vi "ke37xx Channel Write.vi"(0 "VISA Resource Name":refnum<visa-resource-name>, 5 "Channel":string, 7 "Data (0)":string="0", 9 "Width (1)":string="1", 11 "error in (no error)":errorcluster) -> (4 "VISA Resource Name Out":refnum<visa-resource-name>, 15 "error out":errorcluster)   [LabVIEW 2009, in "Keithley 3700 Series.lvlib"]
doc: "This VI provides a way to write data to Digital I/O, Totalizer and DAC channels."
uses:
  <instrlib>/Keithley 3706/Keithley 3700 Series.lvlib
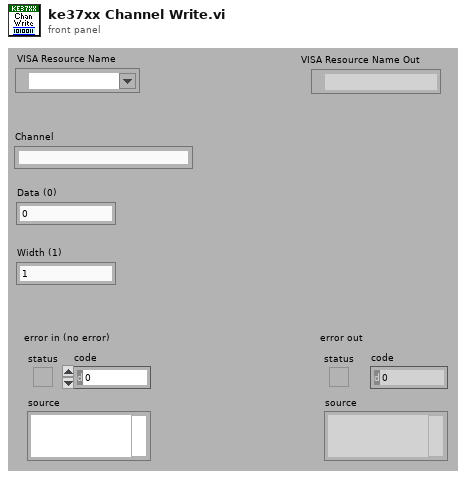
[diagram p1: front panel]
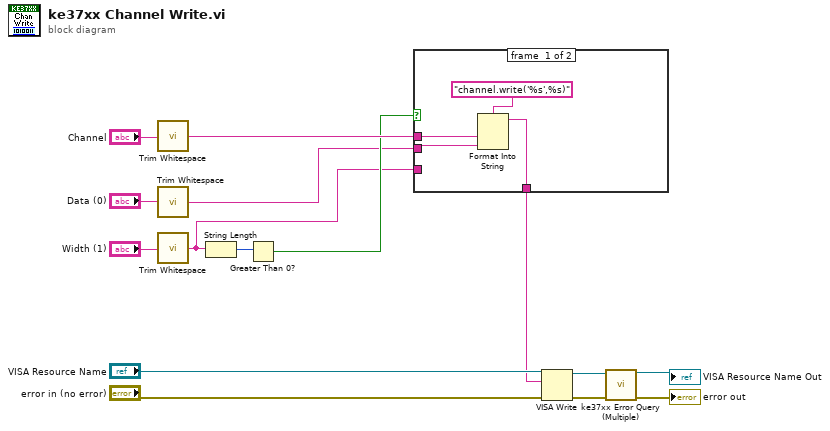
[diagram p0: block diagram]
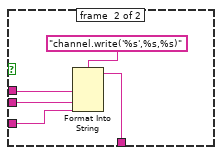
[diagram p2: hidden frame]
diagram:
  n1 = call <vilib>:"Trim Whitespace.vi"("string"="Channel") -> ("trimmed string"=w9:string)  [unwired: 1 in]
  n2 = call <vilib>:"Trim Whitespace.vi"("string"="Data (0)") -> ("trimmed string"=w2:string)  [unwired: 1 in]
  n3 = call <vilib>:"Trim Whitespace.vi"("string"="Width (1)") -> ("trimmed string"=w1:string)  [unwired: 1 in]
  n4 = String Length(string=w1) -> (length=w6:i32)
  n5 = Greater Than 0?(x=w6) -> (x > 0?=w4:bool)
  n6 = case shown="False" w4 {
    tunnel: [w18 w22] -> w11
    tunnel: w9 -> [w17 w23]
    tunnel: w2 -> [w16 w21]
    tunnel: w1 -> [_ w20]
    frame #0 {
      n7 = Format Into String(format string="channel.write('%s',%s)", w17, w16) -> (resulting string=w18:string)  [unwired: 2 in, 1 out]
    }
    frame #1 {
      n8 = Format Into String(format string="channel.write('%s',%s,%s)", w23, w21, w20) -> (resulting string=w22:string)  [unwired: 2 in, 1 out]
    }
  }
  n9 = VISA Write(VISA resource name="VISA Resource Name", write buffer=w11, error in (no error)="error in (no error)") -> (VISA resource name out=w8:refnum<visa-resource-name>, error out=w7:errorcluster)  [unwired: 1 out]
  n10 = call <instrlib>:"ke37xx Error Query (Multiple).vi"("VISA resource name"=w8, "error in (no error)"=w7) -> ("VISA resource name out"=→"VISA Resource Name Out":refnum<visa-resource-name>, "error out"=→"error out":errorcluster)  [unwired: 12 out]
